vi "VGD ECL AHMI PF SubVI05.vi"(8 "error in":errorcluster, 11 "FRONTAL":T1) -> ()   [LabVIEW 2020]
uses:
  <vilib>/vision/Image Controls.llb/IMAQ Image.ctl
  <vilib>/vision/Contour.llb/IMAQ Contour Curve Extraction.ctl
  <vilib>/vision/Measure.llb/Edge Options.ctl
  <vilib>/vision/Measure.llb/Edge Polarity.ctl
  <vilib>/vision/NI_Vision_Development_Module.lvlib
panel:
  out "Linearidad":dbl[](array[numeric])
  out "Image 5":T1(plugin-control)
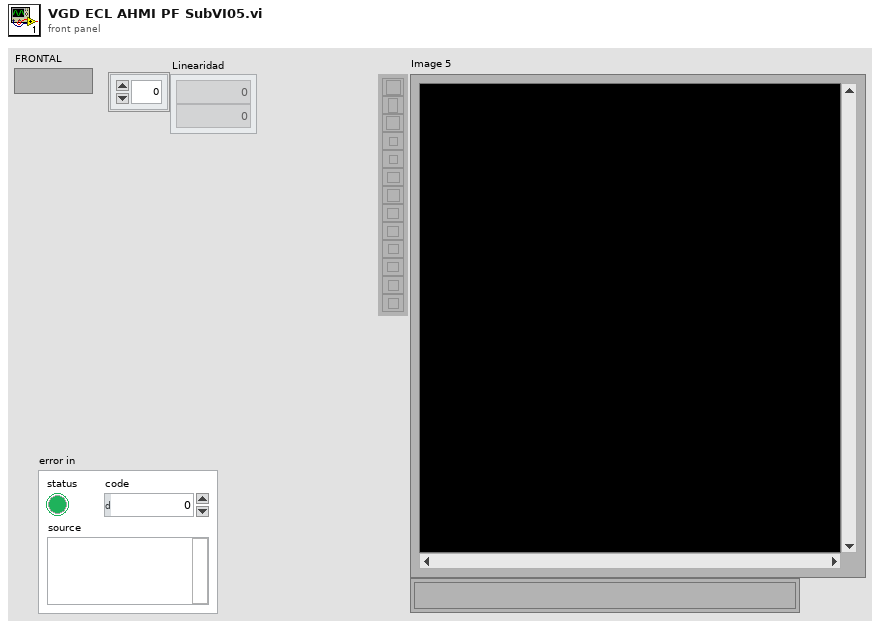
[diagram p1: front panel]
types:
  T1 = typedef "IMAQ Image.ctl" = refnum<image>
  T2 = cluster{"Overlay?":bool, "Color":u32, "Width":u32, "Maintain Width?":bool}
  T3 = typedef "IMAQ Contour Curve Extraction.ctl" = cluster{"Extraction Mode":u32, "Edge Threshold":i32, "Edge Filter Size":u32, "Min Length":i32, "Search Step Size":i32, "Max Endpoint Gap":i32, "Subpixel":bool}
  T4 = enum16{"Closest To Search Start", "Maximum Length", "Strongest Mean Gradient Change"}
  T5 = enum16{"Rect Left To Right", "Rect Right To Left", "Rect Top To Bottom", "Rect Bottom To Top", "Annulus Inner To Outer", "Annulus Outer To Inner", "Annulus Start Angle To End Angle", "Annulus End Angle To Start Angle"}
  T6 = typedef "IMAQ Rectangle" = cluster{"Left":i32, "Top":i32, "Right":i32, "Bottom":i32, "Rotation":dbl}
  T7 = cluster{"Left":i32, "Top":i32, "Right":i32, "Bottom":i32}
  T8 = typedef "Image Type" = u32
  T9 = typedef "ROI Descriptor" = cluster{"Global Rectangle":i32[], "Contours":cluster{"ID":enum32{"External", "Internal"}, "Type":u32, "Coordinates":i32[]}[]}
  T10 = typedef "Edge Options.ctl" = cluster{"Edge Polarity":T11, "Kernel Size":u32, "Width":u32, "Minimum Edge Strength":sgl, "Interpolation Type":enum32{"Zero Order", "Bilinear", "Quadratic", "Cubic", "Bilinear Fixed"}, "Data Processing Method":enum32{"Average", "Median"}}
  T11 = typedef "Edge Polarity.ctl" = u32
  T12 = cluster{"Search Direction":u32, "Edge Options":T10, "Show Search Area":bool, "Show Search Lines":bool, "Show Edges Found":bool, "Show Result":bool, "Search Area Color":u32, "Search Lines Color":u32, "Edge Locations Color":u32, "Result Color":u32, "Overlay Group Name":string}
  T13 = cluster{"Point1 (Pixels)":cluster{"X":sgl, "Y":sgl}, "Point2 (Pixels)":cluster{"X":sgl, "Y":sgl}, "Point1 (Real-World)":cluster{"X":sgl, "Y":sgl}, "Point2 (Real-World)":cluster{"X":sgl, "Y":sgl}, "Angle (Pixel)":dbl, "Angle (Real-World)":dbl, "Score":dbl, "Straightness":dbl, "Average SNR (db)":dbl, "Calibration Valid":bool}[]
  T14 = cluster{"Point1 (Pixels)":cluster{"X":sgl, "Y":sgl}, "Point2 (Pixels)":cluster{"X":sgl, "Y":sgl}, "Point1 (Real-World)":cluster{"X":sgl, "Y":sgl}, "Point2 (Real-World)":cluster{"X":sgl, "Y":sgl}, "Angle (Pixel)":dbl, "Angle (Real-World)":dbl, "Score":dbl, "Straightness":dbl, "Average SNR (db)":dbl, "Calibration Valid":bool}
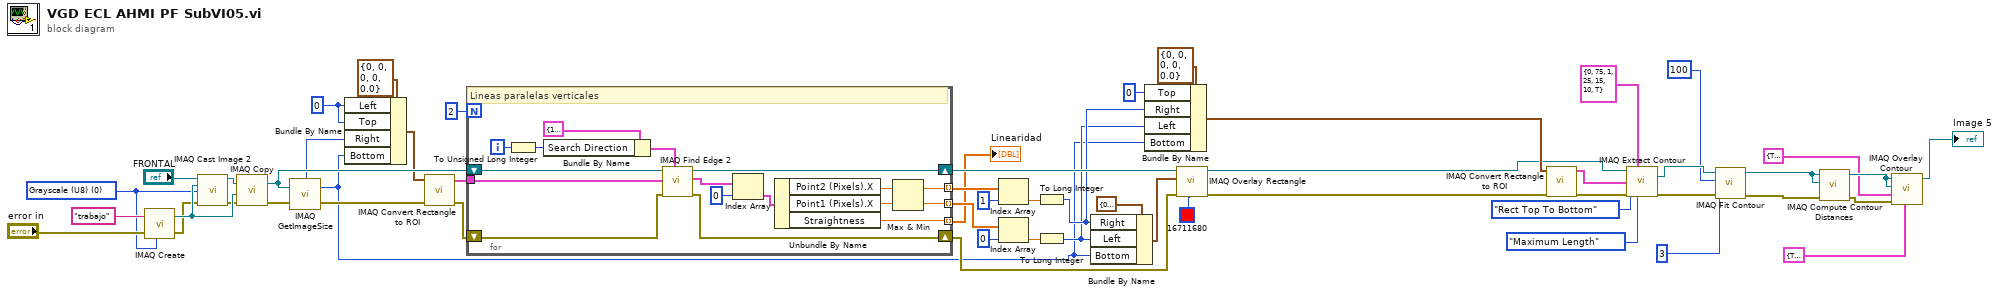
[diagram p0: block diagram]
diagram:
  w41 = 0 ("Left")
  w48 = T8 0 items=["Grayscale (U8)", "Grayscale (I16)", "Grayscale (SGL)", "Complex (CSG)", "RGB (U32)", "HSL (U32)", "RGB (U64)", "Grayscale (U16)"] ("Image Type")
  n1 = call "IMAQ Create"("Image Name"="trabajo", "Image Type"=w48, "error in (no error)"="error in") -> ("New Image"=w50:T1, "error out"=w46:errorcluster)  [unwired: 2 in]
  n2 = call "IMAQ Cast Image 2"("Image Src"="FRONTAL", "Image Dst"=w50, "Image Type"=w48, "error in (no error)"=w46) -> ("Image Dst Out"=w53:T1, "error out"=w49:errorcluster)  [unwired: 10 in]
  n3 = call "IMAQ Copy"("error in (no error)"=w49, "Image Dst"=w50, "Image Src"=w53) -> ("error out"=w45:errorcluster, "Image Dst Out"=w43:T1)  [unwired: 3 in]
  n4 = call "IMAQ GetImageSize"("Image"=w43, "error in (no error)"=w45) -> ("Y Resolution"=w21:i32, "X Resolution"=w40:i32, "error out"=w44:errorcluster)  [unwired: 2 in]
  n5 = Bundle By Name(cluster=T6 {"Left"=0, "Top"=0, "Right"=0, "Bottom"=0, "Rotation"=0.0} ("Rectangle"), "Left"=w41, "Top"=w41, "Right"=w40, "Bottom"=w21) -> (w32:T6)
  n6 = call "IMAQ Convert Rectangle to ROI"("error in (no error)"=w44, "Rectangle"=w32) -> ("error out"=w47:errorcluster, "ROI Descriptor"=w39:T9)  [unwired: 7 in]
  n7 = for {
    N: 2 -> [_]
    shift-right: [w68] -> w31
    shift-left: w43 -> [w71]
    tunnel: [w61] -> w36 mode=indexing
    tunnel: [w60] -> w38 mode=indexing
    tunnel: w39 -> [w58]
    shift-right: [w56] -> w28
    shift-left: w47 -> [w59]
    tunnel: [w55] -> w9 mode=indexing
    i -> [w67]
    # "Lineas paralelas verticales"
    n8 = To Unsigned Long Integer(number=w67) -> (unsigned 32bit integer=w57:u32)
    n9 = Bundle By Name(cluster=T12 {"Search Direction"=1, "Edge Options"={"Edge Polarity"=0, "Kernel Size"=3, "Width"=3, "Minimum Edge Strength"=10.0, "Interpolation Type"=enum."Bilinear Fixed", "Data Processing Method"=enum."Average"}, "Show Search Area"=FALSE, "Show Search Lines"=FALSE, "Show Edges Found"=FALSE, "Show Result"=FALSE, "Search Area Color"=65280, "Search Lines Color"=255, "Edge Locations Color"=16776960, "Result Color"=16711680, "Overlay Group Name"=""} ("Options"), "Search Direction"=w57) -> (w69:T12)
    n10 = call "IMAQ Find Edge 2"("Options"=w69, "error in (no error)"=w59, "ROI Descriptor"=w58, "Image"=w71) -> ("error out"=w56:errorcluster, "Straight Edges"=w66:T13, "Image Out"=w68:T1)  [unwired: 4 in, 1 out]
    n11 = Index Array(array=w66, index=0) -> (element=w64:T14)
    n12 = Unbundle By Name(w64) -> ("Point2 (Pixels).X"=w62:sgl, "Point1 (Pixels).X"=w63:sgl, "Straightness"=w55:dbl)
    n13 = Max & Min(x=w62, y=w63) -> (max(x,y)=w60:sgl, min(x,y)=w61:sgl)
  }
  "Linearidad" <- w9
  n14 = Index Array(array=w38, index=1) -> (element=w33:sgl)
  n15 = Index Array(array=w36, index=0) -> (element=w34:sgl)
  n16 = To Long Integer(number=w33) -> (32bit integer=w23:i32)
  n17 = To Long Integer(number=w34) -> (32bit integer=w22:i32)
  n18 = Bundle By Name(cluster=T7 {"Left"=0, "Top"=0, "Right"=0, "Bottom"=0} ("Rectangle"), "Right"=w23, "Left"=w22, "Bottom"=w21) -> (w29:T7)
  n19 = Bundle By Name(cluster=T6 {"Left"=0, "Top"=0, "Right"=0, "Bottom"=0, "Rotation"=0.0} ("Rectangle"), "Top"=0, "Right"=w23, "Left"=w22, "Bottom"=w21) -> (w19:T6)
  n20 = call "IMAQ Overlay Rectangle"("Color"=u32 16711680, "error in (no error)"=w28, "Rectangle"=w29, "Image"=w31) -> ("error out"=w20:errorcluster, "Image Out"=w17:T1)  [unwired: 6 in]
  n21 = call "IMAQ Convert Rectangle to ROI"("error in (no error)"=w20, "Rectangle"=w19) -> ("error out"=w18:errorcluster, "ROI Descriptor"=w16:T9)  [unwired: 7 in]
  n22 = call "IMAQ Extract Contour"("Source Image"=w17, "Curve Extraction"=T3 {"Extraction Mode"=0, "Edge Threshold"=75, "Edge Filter Size"=1, "Min Length"=25, "Search Step Size"=15, "Max Endpoint Gap"=10, "Subpixel"=TRUE}, "ROI Descriptor"=w16, "Search Direction"=T5."Rect Top To Bottom", "error in (no error)"=w18, "Contour Selection"=T4."Maximum Length") -> ("Contour Image Out"=w10:T1, "error out"=w12:errorcluster)  [unwired: 5 in, 3 out]
  n23 = call-poly "IMAQ Fit Contour"("error in (no error)"=w12, "Degree"=u32 3, "Control Points"=u32 100, "Contour Image"=w10) -> ("error out"=w5:errorcluster, "Contour Image Out"=w6:T1)  [unwired: 6 out]
  n24 = call "IMAQ Compute Contour Distances"("error in (no error)"=w5, "Template Contour Image"=w6, "Target Contour Image"=w6) -> ("error out"=w4:errorcluster, "Target Contour Image Out (dup)"=w3:T1)  [unwired: 2 in, 5 out]
  n25 = call "IMAQ Overlay Contour"("Contour Equation Settings"=T2 {"Overlay?"=TRUE, "Color"=3381759, "Width"=1, "Maintain Width?"=TRUE}, "error in (no error)"=w4, "Contour Points Settings"=T2 {"Overlay?"=TRUE, "Color"=6618880, "Width"=1, "Maintain Width?"=TRUE}, "Contour Image"=w3, "Image"=w3) -> ("Image Out"=→"Image 5":T1)  [unwired: 1 in, 5 out]
